vi "Set Frequency.vi"() -> ()   [LabVIEW 2015, in "Monitoring_receiver.lvlib"]
uses:
  Monitoring_receiver.lvlib
panel:
  out "msg.sent":string
  out "Freq":dbl format="%#_6p"
  in  "OK Button":bool
  in  "Freq (Hz)":dbl step=1000.0 format="%#_6f"
  in  "Server Closed":string="The server VI closed the connection."
  in  "Stop":bool
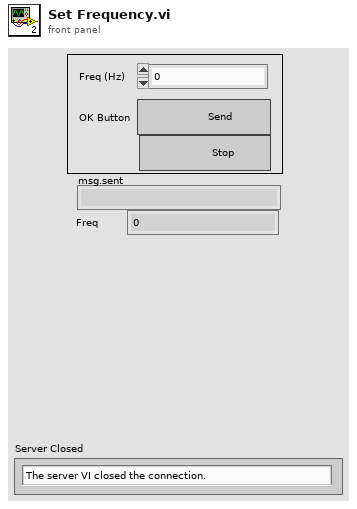
[diagram p1: front panel]
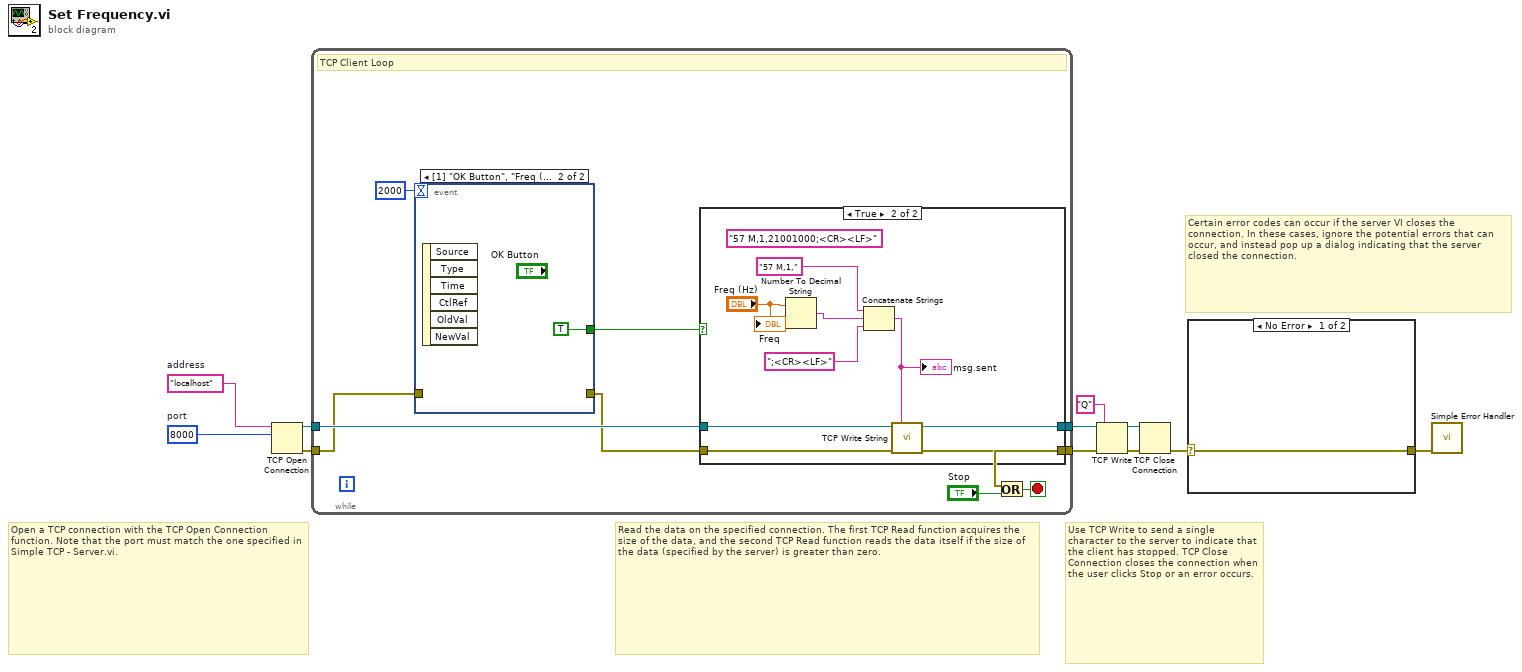
[diagram p0: block diagram]
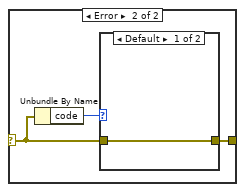
[diagram p2: hidden frame]
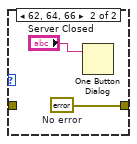
[diagram p3: hidden frame]
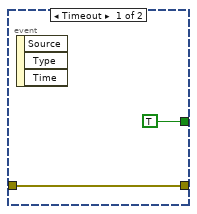
[diagram p4: hidden frame]
diagram:
  w1 = u16 8000  # port
  w2 = "localhost"  # address
  # "Certain error codes can occur if the server VI closes the connection. In these cases, ignore the potential errors that can occur, and instead pop up a dialog indicating that the server closed the connection."
  # "Use TCP Write to send a single character to the server to indicate that the client has stopped. TCP Close Connection closes the connection when the user clicks Stop or an error occurs."
  # "Read the data on the specified connection. The first TCP Read function acquires the size of the data, and the second TCP Read function reads the data itself if the size of the data (specified by the server) is greater than zero."
  # "Open a TCP connection with the TCP Open Connection function. Note that the port must match the one specified in Simple TCP - Server.vi."
  n1 = TCP Open Connection(address=w2, remote port or service name=w1) -> (connection ID=w11:refnum<k5>, error out=w10:errorcluster)  [unwired: 3 in]
  n2 = while {
    tunnel: w10 -> [w15]
    tunnel: w11 -> [w18]
    tunnel: [w17] -> w8
    tunnel: [w16] -> w6
    stop <- w19 stop-if-true
    # "TCP Client Loop"
    n3 = event shown="[1] \"OK Button\", \"Freq (Hz)\": Key Repeat" {
      selector: _ -> [_ _]
      dyn-events: _ -> [_ _]
      timeout: 2000 -> [_ _]
      tunnel: w15 -> [w22 _]
      tunnel: [w22 _] -> w14
      tunnel: [TRUE TRUE] -> w13
      event Timeout {
        n4 = event-data() -> ()  [unwired: 1 in, 3 out]
      }
      event "OK Button", "Freq (Hz)": Value Change {
        n5 = event-data() -> ()  [unwired: 1 in, 6 out]
      }
    }
    n6 = case shown="True" w13 {
      tunnel: w18 -> [w24 w29]
      tunnel: w14 -> [w25 w28]
      tunnel: [w24 w27] -> w17
      tunnel: [w25 w26] -> w16
      frame False {
      }
      frame True {
        (unwired) "57 M,1,21001000;<CR><LF>"
        n7 = Number To Decimal String(number="Freq (Hz)") -> (decimal integer string=w31:string)  [unwired: 1 in]
        n8 = Concatenate Strings("57 M,1,", w31, ";<CR><LF>") -> (w30:string)
        "msg.sent" <- w30
        n9 = call <vilib>:"TCP Write String.vi"("error in (no error)"=w28, "data in"=w30, "connection ID"=w29) -> ("error out"=w26:errorcluster, "connection ID out"=w27:refnum<k5>)  [unwired: 7 in]
        "Freq" <- "Freq (Hz)"
      }
    }
    n10 = Or(x=w16, y="Stop") -> (x .or. y?=w19:bool)
  }
  n11 = TCP Write(connection ID=w8, data in="Q", error in (no error)=w6) -> (connection ID out=w9:refnum<k5>, error out=w7:errorcluster)  [unwired: 2 out]
  n12 = TCP Close Connection(connection ID=w9, error in (no error)=w7) -> (error out=w4:errorcluster)  [unwired: 1 in, 1 out]
  n13 = case shown="No Error" w4 {
    selector: w4 -> [w35 w37]
    tunnel: [w35 w36] -> w3
    frame No Error {
    }
    frame Error {
      n14 = Unbundle By Name(w37) -> ("code"=w38:i32)
      n15 = case shown="Default" w38 {
        tunnel: w37 -> [w39 _]
        tunnel: [w39 w41] -> w36
        frame Default {
        }
        frame 62, 64, 66 {
          w41 = errorcluster {"status"=FALSE, "code"=0, "source"=""}  # No error
          n16 = One Button Dialog(message="Server Closed") -> ()  [unwired: 1 in, 1 out]
        }
      }
    }
  }
  n17 = call <vilib>:"Simple Error Handler.vi"("error in (no error)"=w3) -> ()  [unwired: 4 in, 5 out]
